vi "Test Create Logger with File Sink.vi"(11 "Test Case In":refnum<class "File Sink.lvclass">) -> (0 "error out":errorcluster, 3 "Test Case Out":refnum<class "File Sink.lvclass">)   [LabVIEW 2020, in "File Sink.lvclass"]
uses:
  File Sink.lvclass
  C:/Program Files (x86)/National Instruments/LabVIEW 2020/vi.lib/Astemes/LUnit/Test Case.lvclass
  Source/Type Defs/Debug Level.ctl
  <vilib>/Astemes/LUnit/Test Case.lvclass/Test Case.ctl
  8e009b1c-5ae2-41f0-bb19-d33c7d52fc0a.vi
  494f9ffb-8588-4f0b-9448-a169cb2ac2eb.vi
  63f58c3f-d290-4083-b4f7-4fb5527ed70c.vi
  <vilib>/Astemes/LUnit/Core/LUnit Test Case/Private/Append Fail Result.vi
  <vilib>/Astemes/LUnit/Core/LUnit Test Case/Private/Append Pass Result.vi
  8e009b1c-5ae2-41f0-bb19-d33c7d52fc0a.vi/9c5d11cd-9439-4240-a1ee-d9baace9c924.vi
  494f9ffb-8588-4f0b-9448-a169cb2ac2eb.vi/9c5d11cd-9439-4240-a1ee-d9baace9c924.vi
  63f58c3f-d290-4083-b4f7-4fb5527ed70c.vi/9c5d11cd-9439-4240-a1ee-d9baace9c924.vi
  <vilib>/Astemes/LUnit/Core/LUnit Test Case/Private/Run In UI.vi
  <vilib>/Utility/error.llb/Clear Errors.vi
  Source/Sinks/File Sink/File Sink.lvclass
  C:/Users/hughe_cx/Documents/05_repos/LVLog/Source/Sinks/Sink/Sink.lvclass
  Source/LV Log.lvlib
  Source/Logger/Logger.lvclass
  <vilib>/Astemes/LUnit/Test Case.lvclass
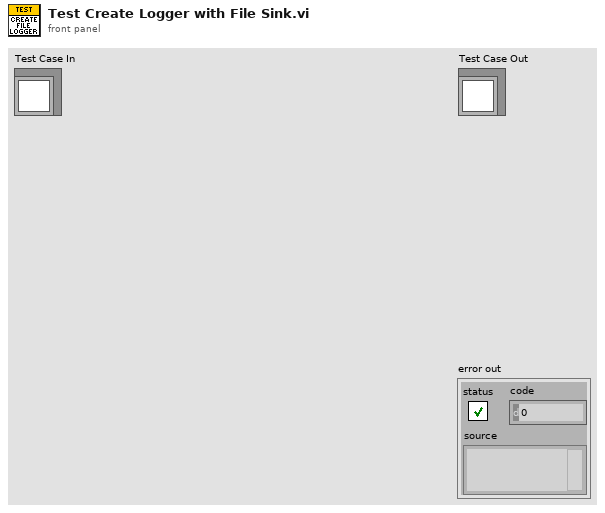
[diagram p1: front panel]
types:
  T1 = typedef "LV Log.lvlib/Debug Level.ctl" = enum16{"DEFAULT", "DEBUG", "INFO", "WARN", "ERROR", "FATAL"}
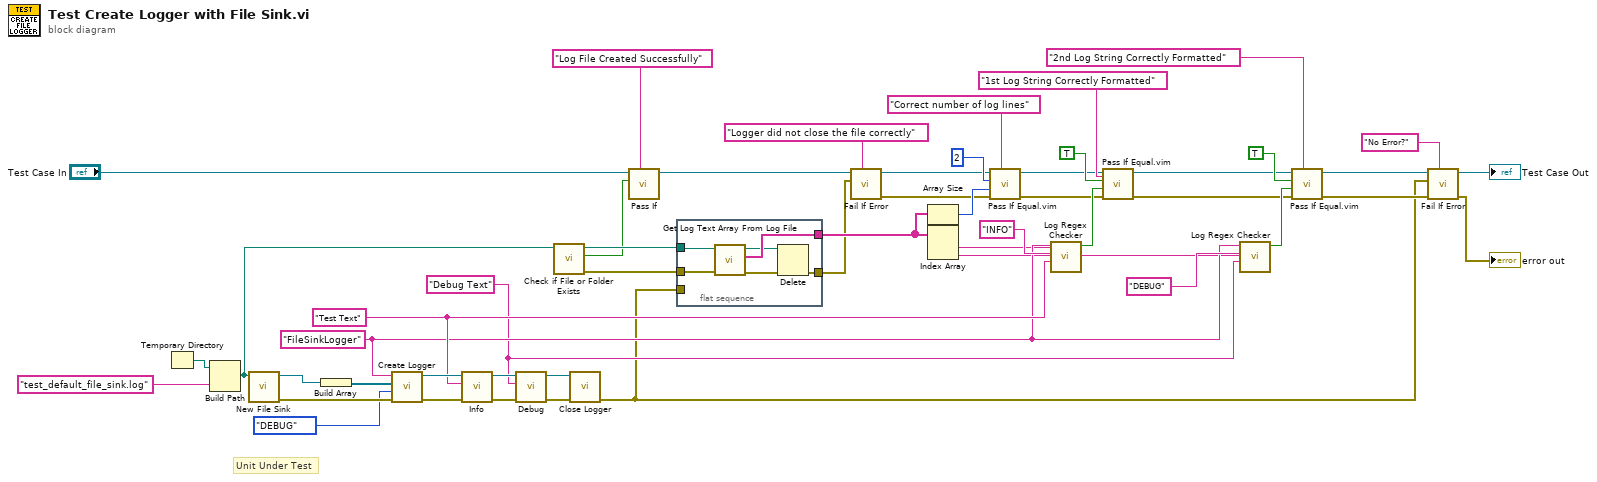
[diagram p0: block diagram]
diagram:
  w36 = "Debug Text" ("Log Text")
  w45 = "Test Text" ("Log Text")
  w37 = "FileSinkLogger" ("Name")
  # "Unit Under Test"
  n1 = Temporary Directory() -> (w50:path)
  n2 = Build Path(base path=w50, name or relative path="test_default_file_sink.log" ("format string")) -> (appended path=w23:path)
  n3 = call "New File Sink.vi"("File Path"=w23) -> ("error out"=w19:errorcluster, "File Sink out"=w18:refnum<class "File Sink.lvclass">)  [unwired: 9 in]
  n4 = Build Array(w18) -> (w17:refnum<class "File Sink.lvclass">[])
  n5 = call "Create Logger.vi"("error in (no error)"=w19, "Debug Level (Default)"=Debug_Level."DEBUG" ("Debug Level in"), "Sinks (Default)"=w17, "Name"=w37) -> ("error out"=w49:errorcluster, "Logger out"=w48:refnum<class "Logger.lvclass">)  [unwired: 6 in]
  n6 = call "Info.vi"("error in (no error)"=w49, "Log Text"=w45, "Logger in"=w48) -> ("error out"=w44:errorcluster, "Logger out"=w43:refnum<class "Logger.lvclass">)  [unwired: 6 in, 1 out]
  n7 = call "Debug.vi"("error in (no error)"=w44, "Log Text"=w36, "Logger in"=w43) -> ("error out"=w12:errorcluster, "Logger out"=w11:refnum<class "Logger.lvclass">)  [unwired: 6 in, 1 out]
  n8 = call <vilib>:"Check if File or Folder Exists.vi"("path"=w23) -> ("error out"=w22:errorcluster, "file or folder exists?"=w21:bool, "dup path"=w24:path)  [unwired: 8 in]
  n9 = call "Close Logger.vi"("error in (no error)"=w12, "Logger in"=w11) -> ("error out"=w10:errorcluster)  [unwired: 9 in]
  n10 = call <vilib>:"Pass If.vi"("Description"="Log File Created Successfully", "Pass?"=w21, "LUnit Test Case In"="Test Case In") -> ("LUnit Test Case Out"=w7:refnum<class "File Sink.lvclass">)  [unwired: 7 in, 1 out]
  n11 = flat-sequence {
    tunnel: w24 -> [w56]
    tunnel: [w55] -> w30
    tunnel: w22 -> [w52]
    tunnel: w10 -> [_]
    tunnel: [w51] -> w3
    frame #0 {
      n12 = call "Get Log Text Array From Log File.vi"("error in"=w52, "Log File Path in"=w56) -> ("error out"=w54:errorcluster, "Log Text Array"=w55:string[], "Log File Path out"=w53:path)  [unwired: 7 in]
      n13 = Delete(path (use dialog)=w53, error in=w54) -> (error out=w51:errorcluster)  [unwired: 3 in, 2 out]
    }
  }
  n14 = call <vilib>:"Fail If Error.vi"("Description"="Logger did not close the file correctly", "Assert error"=w3, "LUnit Test Case In"=w7) -> ("error out"=w4:errorcluster, "LUnit Test Case Out"=w6:refnum<class "File Sink.lvclass">)  [unwired: 7 in]
  n15 = Array Size(array=w30) -> (size(s)=w29:i32)
  n16 = Index Array(array=w30) -> (element #1=w35:string, element #2=w34:string)  [unwired: 2 in]
  n17 = call "Pass If Equal.vim"("Description"="Correct number of log lines", "error in (no error)"=w4, "Actual"=w29, "Expected"=2, "LUnit Test Case In"=w6) -> ("error out"=w25:errorcluster, "LUnit Test Case Out"=w31:refnum<class "File Sink.lvclass">)  [unwired: 5 in]
  n18 = call "Log Regex Checker.vi"("Log String"=w35, "Expected Log Text (Any)"=w45, "Expected Log Level (Any)"="INFO", "Expected Logger Name (Any)"=w37) -> ("Math Found"=w41:bool)  [unwired: 5 in, 2 out]
  n19 = call "Pass If Equal.vim"("Description"="1st Log String Correctly Formatted", "error in (no error)"=w25, "Actual"=w41, "Expected"=TRUE, "LUnit Test Case In"=w31) -> ("error out"=w26:errorcluster, "LUnit Test Case Out"=w33:refnum<class "File Sink.lvclass">)  [unwired: 5 in]
  n20 = call "Log Regex Checker.vi"("Log String"=w34, "Expected Log Text (Any)"=w36, "Expected Log Level (Any)"="DEBUG", "Expected Logger Name (Any)"=w37) -> ("Math Found"=w40:bool)  [unwired: 5 in, 2 out]
  n21 = call "Pass If Equal.vim"("Description"="2nd Log String Correctly Formatted", "error in (no error)"=w26, "Actual"=w40, "Expected"=TRUE, "LUnit Test Case In"=w33) -> ("error out"=w27:errorcluster, "LUnit Test Case Out"=w32:refnum<class "File Sink.lvclass">)  [unwired: 5 in]
  n22 = call <vilib>:"Fail If Error.vi"("Description"="No Error?", "error in (no error)"=w27, "Assert error"=w10, "LUnit Test Case In"=w32) -> ("error out"=→"error out":errorcluster, "LUnit Test Case Out"=→"Test Case Out":refnum<class "File Sink.lvclass">)  [unwired: 6 in]
